vi "Lbb_2024.vi"(3 "Gamma_w":dbl, 4 "d^2Bw(T)/dT^2":dbl, 5 "dBw(T)/dT":dbl, 6 "Bw(T)":dbl, 7 "Gamma_dryair":dbl, 8 "d^2Bd(T)/dT^2":dbl, 9 "dBd(T)/dT":dbl, 10 "Bd(T)":dbl, 11 "Temperature [K]":dbl) -> (0 "Lbbw":dbl, 1 "Lbbd":dbl)   [LabVIEW 2016]
uses:
  2022/SOS_Global_2022.vi
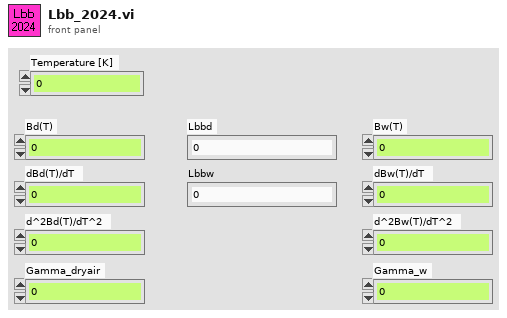
[diagram p1: front panel]
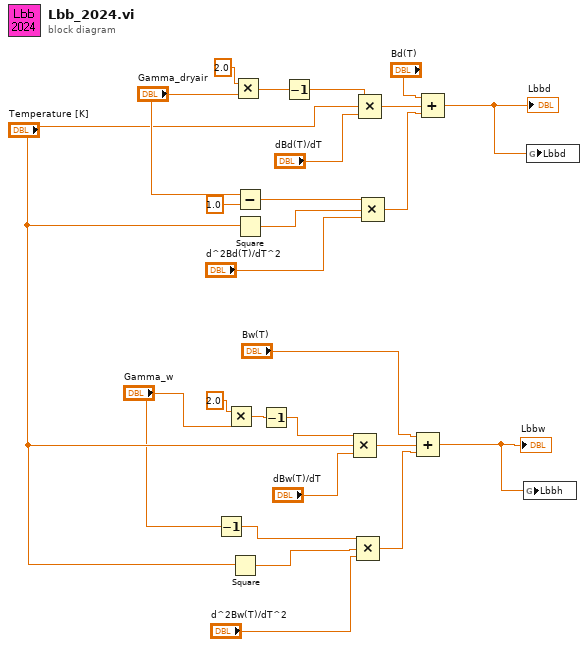
[diagram p0: block diagram]
diagram:
  n1 = Decrement(x="Gamma_w") -> (x-1=w1:dbl)
  n2 = Multiply(x=2.0, y="Gamma_w") -> (x*y=w4:dbl)
  n3 = Square(x="Temperature [K]") -> (x^2=w12:dbl)
  n4 = Multiply(x=2.0, y="Gamma_dryair") -> (x*y=w25:dbl)
  n5 = Subtract(x="Gamma_dryair", y=1.0) -> (x-y=w21:dbl)
  n6 = Square(x="Temperature [K]") -> (x^2=w19:dbl)
  n7 = Decrement(x=w4) -> (x-1=w3:dbl)
  n8 = Decrement(x=w25) -> (x-1=w5:dbl)
  n9 = Compound Arithmetic op=MULTIPLY(w3, "Temperature [K]", "dBw(T)/dT") -> (w11:dbl)
  n10 = Compound Arithmetic op=MULTIPLY(w1, w12, "d^2Bw(T)/dT^2") -> (w10:dbl)
  n11 = Compound Arithmetic op=MULTIPLY(w5, "Temperature [K]", "dBd(T)/dT") -> (w18:dbl)
  n12 = Compound Arithmetic op=MULTIPLY(w21, w19, "d^2Bd(T)/dT^2") -> (w17:dbl)
  n13 = Compound Arithmetic op=ADD("Bw(T)", w11, w10) -> (w6:dbl)
  "Lbbw" <- w6
  n14 = Compound Arithmetic op=ADD("Bd(T)", w18, w17) -> (w7:dbl)
  "Lbbd" <- w7
  n15 = global write "SOS_Global_2022.vi" "Lbbh"(w6) -> ()
  n16 = global write "SOS_Global_2022.vi" "Lbbd"(w7) -> ()
